vi "Populate Control Labels.vi"(8 "error in (no error)":errorcluster, 10 "Ordered Controls":refnum<vi>[](array[refnum]), 11 "Controls in":variant) -> (0 "error out":errorcluster, 2 "UIDs":i32[](array[numeric]), 3 "Controls out":variant)   [LabVIEW 2014]
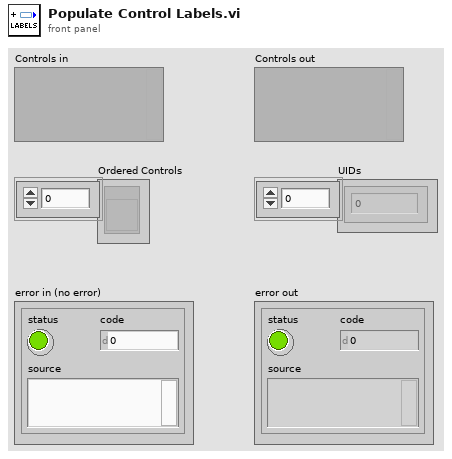
[diagram p1: front panel]
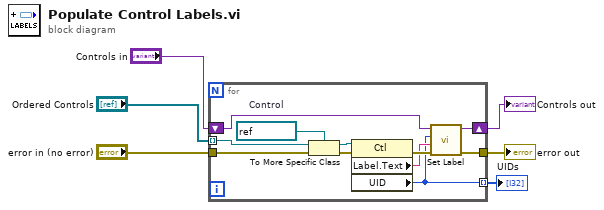
[diagram p0: block diagram]
diagram:
  n1 = for {
    tunnel: "Ordered Controls" -> [w14] mode=indexing
    shift-right: [w11] -> w6
    shift-left: "Controls in" -> [w12]
    tunnel: "error in (no error)" -> [w13]
    tunnel: [w9] -> w2
    tunnel: [w7] -> w1 mode=indexing
    w17 = refnum<vi> refnum  # Control
    n2 = To More Specific Class(target class=w17, reference=w14, error in=w13) -> (specific class reference=w16:refnum<vi>, error out=w15:errorcluster)
    n3 = property class="Ctl"(reference=w16, error in=w15) -> (error out=w10:errorcluster, "Label.Text"=w8:string, "UID"=w7:i32)  [unwired: 1 out]
    n4 = call "Set Label.vi"("Error In"=w10, "Label"=w8, "UID"=w7, "Controls"=w12) -> ("Error Out"=w9:errorcluster, "Controls"=w11:variant)  [unwired: 6 in]
  }
  "Controls out" <- w6
  "error out" <- w2
  "UIDs" <- w1
